vi "Load Data.vi"(8 "error in (no error)":errorcluster caption="错误输入（无错误）", 11 "Node*":refnum<data-value>) -> (0 "error out":errorcluster caption="错误输出", 2 "Display Config":T1={"Display Mode"=enum."时域", "ChTag[]"=[], "window"=1, "Range"={"Minimum"=0.0, "Maximum"=0.0, "Increment"=0.0, "Minor Increment"=0.0, "Start"=0.0}} {"window" items=["矩形"=0, "Hanning"=1, "Hamming"=2, "Blackman-Harris"=3, "Exact Blackman"=4, "Blackman"=5, "Flat Top"=6, "4阶Blackman-Harris "=7, "7阶Blackman-Harris"=8, "Low Sidelobe"=9, "Blackman Nuttall"=11, "三角"=30, "Bartlett-Hanning"=31, "Bohman"=32, "Parzen"=33, "Welch"=34, "Kaiser"=60, "Dolph-Chebyshev"=61, "高斯"=62]})   [LabVIEW 2016]
uses:
  PCM PanelSplit.lvclass
  Display Mode.ctl
  <vilib>/Analysis/4window.llb/windowTd.ctl
  <vilib>/Analysis/NI_AALPro.lvlib
  <vilib>/Utility/miscctls.llb/LVRangeTypeDef.ctl
  Display Config.ctl
  PanelSplitToolkit/PanelObject/PanelObject.lvclass
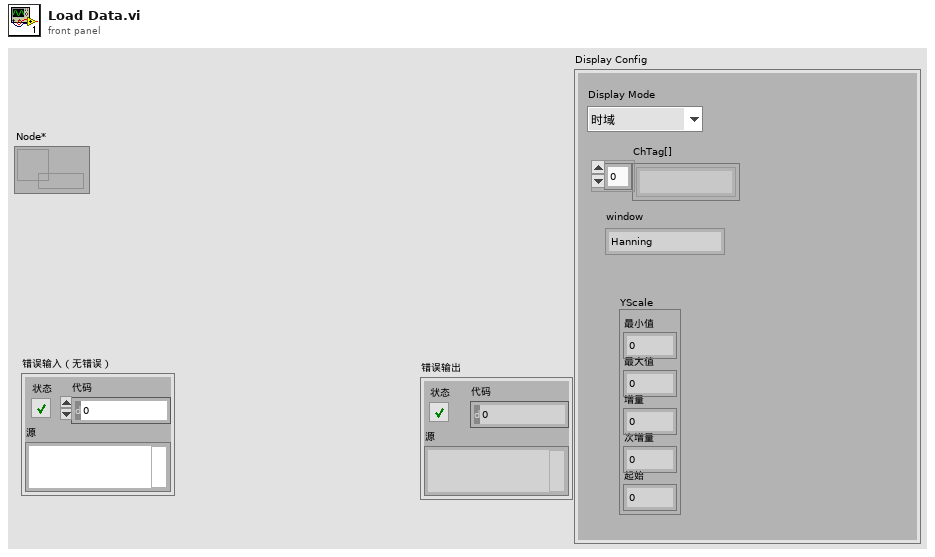
[diagram p1: front panel]
types:
  T1 = typedef "PCM PanelSplit.lvclass/Display Config.ctl" = cluster{"Display Mode":T2, "ChTag[]":string[], "window":T3, "Range":T4}
  T2 = typedef "PCM PanelSplit.lvclass/Display Mode.ctl" = enum16{"时域", "频谱", "功率谱"}
  T3 = typedef "NI_AALPro.lvlib/windowTd.ctl" = u32
  T4 = typedef "LVRangeTypeDef.ctl" = cluster{"Minimum":dbl, "Maximum":dbl, "Increment":dbl, "Minor Increment":dbl, "Start":dbl}
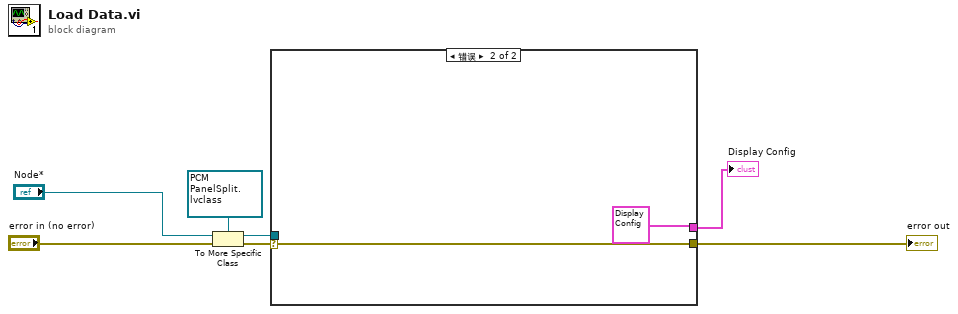
[diagram p0: block diagram]
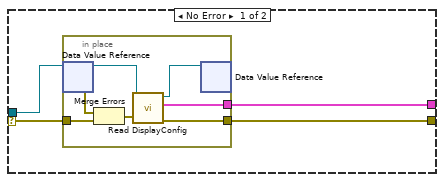
[diagram p2: hidden frame]
diagram:
  n1 = To More Specific Class(target class=refnum<data-value> refnum ("数据值引用"), reference="Node*", error in="error in (no error)") -> (specific class reference=w6:refnum<data-value>, error out=w5:errorcluster)
  n2 = case shown="错误" w5 {
    selector: w5 -> [w10 w20]
    tunnel: w6 -> [w11 _]
    tunnel: [w9 w20] -> w2
    tunnel: [w8 T1 {"Display Mode"=enum."时域", "ChTag[]"=[], "window"=1, "Range"={"Minimum"=0.0, "Maximum"=0.0, "Increment"=0.0, "Minor Increment"=0.0, "Start"=0.0}} ("Display Config")] -> w1
    frame No Error {
      n3 = in-place {
        in-place-border: w10 -> [w13]
        in-place-border: [w16] -> w9
        in-place-border: [w15] -> w8
        n4 = in-place-dvr #1(w11) -> (w18:refnum<class "PCM PanelSplit.lvclass">, w14:errorcluster)
        n5 = Merge Errors(w14, w13) -> (w12:errorcluster)
        n6 = call "Read DisplayConfig.vi"("error in"=w12, "PCM PanelSplit 输入"=w18) -> ("error out"=w16:errorcluster, "Display Config"=w15:T1, "PCM PanelSplit 输出"=w17:refnum<class "PCM PanelSplit.lvclass">)  [unwired: 7 in]
        n7 = in-place-dvr #1(w17) -> ()  [unwired: 2 out]
      }
    }
    frame Error {
    }
  }
  "error out" <- w2
  "Display Config" <- w1
